vi "Event case.vi"() -> ()   [LabVIEW 2019]
panel:
  in  "Forgot Password":bool
  in  "Submit":bool
  in  "Username":string="Atharva"
  in  "Password":string="1234"
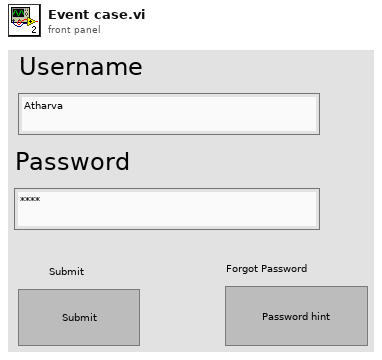
[diagram p1: front panel]
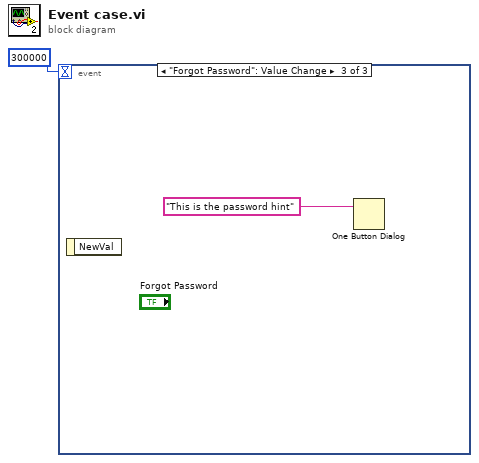
[diagram p0: block diagram]
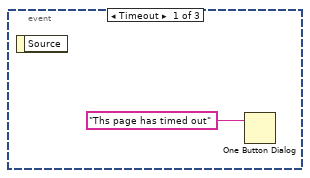
[diagram p2: hidden frame]
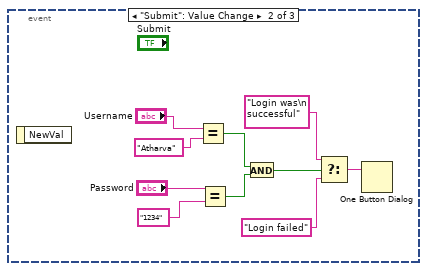
[diagram p3: hidden frame]
diagram:
  n1 = event shown="[2] \"Forgot Password\": Value Change" {
    selector: _ -> [_ _ _]
    dyn-events: _ -> [_ _ _]
    timeout: 300000 -> [_ _ _]
    event Timeout {
      n2 = event-data() -> ()  [unwired: 1 in, 1 out]
      n3 = One Button Dialog(message="Ths page has timed out") -> ()  [unwired: 1 in, 1 out]
    }
    event "Submit": Value Change {
      n4 = event-data() -> ()  [unwired: 1 in, 1 out]
      n5 = Equal?(x="Username", y="Atharva") -> (x = y?=w12:bool)
      n6 = Equal?(x="Password", y="1234") -> (x = y?=w11:bool)
      n7 = And(x=w12, y=w11) -> (x .and. y?=w6:bool)
      n8 = Select(t="Login was\n successful", s=w6, f="Login failed") -> (s? t:f=w3:string)
      n9 = One Button Dialog(message=w3) -> ()  [unwired: 1 in, 1 out]
    }
    event "Forgot Password": Value Change {
      n10 = event-data() -> ()  [unwired: 1 in, 1 out]
      n11 = One Button Dialog(message="This is the password hint") -> ()  [unwired: 1 in, 1 out]
    }
  }
